vi "Setting Zero Point.vi"(6 "Gas Tank":u8, 7 "Count":u8, 9 "output cluster 3":T2 {"Current Settings"."Pump" items=["Pump 0", "Pump 1", "Pump 2", "Pump 3", "Pump 4", "Pump 5"]; "Current Settings"."Chart X axis Timescale" min=20 max=180 step=1; "Current Settings"."RunTime Mode Settings"."Exp. Gas Tank" items=["0.07", "0.031", "0.877", "1.863", "3.881", "5.790", "7.688", "6.000"]; "Current Settings"."RunTime Mode Settings"."Insp. Gas Tank" items=["0.07", "0.031", "0.877", "1.863", "3.881", "5.790", "7.688", "6.000"]; "Current Settings"."RunTime Mode Settings"."I:E Ratio" max=30 scale=0.0..7.0; "Current Settings"."RunTime Mode Settings"."Resp Rate Brpm" min=0 max=30 format="%.2f"; "Current Settings"."TE#2 Configuration"."Serial Port"."XOFF Char" format="%.0x"; "Current Settings"."TE#2 Configuration"."Serial Port"."XON Char" format="%.0x"; "Current Settings"."TE#2 Configuration"."Serial Port"."flow control" items=["None"=0, "XON/XOFF"=1, "RTS/CTS"=2, "DTR/DSR"=4]; "Current Settings"."TE#2 Configuration"."Serial Port"."stop bits" items=["1.0"=10, "1.5"=15, "2.0"=20]; "Current Settings"."TE#2 Configuration"."Serial Port"."data bits" min=5 max=8 step=1; "Current Settings"."TE#2 Configuration"."Serial Port"."baud rate" items=["75"=75, "110"=110, "134"=134, "150"=150, "300"=300, "600"=600, "1200"=1200, "1800"=1800, "2400"=2400, "4800"=4800, "7200"=7200, "9600"=9600, "14400"=14400, "19200"=19200, "28800"=28800, "38400"=38400, "56000"=56000, "57600"=57600, "115200"=115200, "128000"=128000, "230400"=230400]; "Current Settings"."TE#2 Configuration"."Serial Port"."termination char" format="%.0x"; "Current Settings"."TE#1 Configuration"."Serial Port"."XOFF Char" format="%.0x"; "Current Settings"."TE#1 Configuration"."Serial Port"."XON Char" format="%.0x"; "Current Settings"."TE#1 Configuration"."Serial Port"."flow control" items=["None"=0, "XON/XOFF"=1, "RTS/CTS"=2, "DTR/DSR"=4]; "Current Settings"."TE#1 Configuration"."Serial Port"."stop bits" items=["1.0"=10, "1.5"=15, "2.0"=20]; "Current Settings"."TE#1 Configuration"."Serial Port"."data bits" min=5 max=8 step=1; "Current Settings"."TE#1 Configuration"."Serial Port"."baud rate" items=["75"=75, "110"=110, "134"=134, "150"=150, "300"=300, "600"=600, "1200"=1200, "1800"=1800, "2400"=2400, "4800"=4800, "7200"=7200, "9600"=9600, "14400"=14400, "19200"=19200, "28800"=28800, "38400"=38400, "56000"=56000, "57600"=57600, "115200"=115200, "128000"=128000, "230400"=230400]; "Current Settings"."TE#1 Configuration"."Serial Port"."termination char" format="%.0x"; "Current Settings"."Capnometer Configuration"."Device" items=["None", "TidalWave", "LoFlow / Canary", "Capnogard"]; "Current Settings"."Capnometer Configuration"."Serial Port"."XOFF Char" format="%.0x"; "Current Settings"."Capnometer Configuration"."Serial Port"."XON Char" format="%.0x"; "Current Settings"."Capnometer Configuration"."Serial Port"."flow control" items=["None"=0, "XON/XOFF"=1, "RTS/CTS"=2, "DTR/DSR"=4]; "Current Settings"."Capnometer Configuration"."Serial Port"."stop bits" items=["1.0"=10, "1.5"=15, "2.0"=20]; "Current Settings"."Capnometer Configuration"."Serial Port"."data bits" min=5 max=8 step=1; "Current Settings"."Capnometer Configuration"."Serial Port"."baud rate" items=["75"=75, "110"=110, "134"=134, "150"=150, "300"=300, "600"=600, "1200"=1200, "1800"=1800, "2400"=2400, "4800"=4800, "7200"=7200, "9600"=9600, "14400"=14400, "19200"=19200, "28800"=28800, "38400"=38400, "56000"=56000, "57600"=57600, "115200"=115200, "128000"=128000, "230400"=230400]; "Current Settings"."Capnometer Configuration"."Serial Port"."termination char" format="%.0x"; "Current Settings"."DAQx Settings"."Analog Output Settings (Volts)" format="%#.3g"; "Current Settings"."DAQx Settings"."Duty Cycle" min=10.0 max=90.0 format="%.1g"; "Current Settings"."DAQx Settings"."Frequency" min=20.0 max=200.0; "Current Settings"."DataLogging Settings"."Data File Duration (Minutes)" min=2 max=200 format="%#.2g"; "Current Settings"."Calibration Settings"."Tolerance #2" min=2 max=4096; "Current Settings"."Calibration Settings"."Cal. Average" min=2 max=4096; "Current Settings"."Test Settings"."Test Sensor ID" items=["(select)", "RB", "YC", "", "Other"]}, 10 "CalStatus":T1(ring), 11 "output cluster":T10) -> (2 "NewCalStatus":T1(ring), 3 "Count out":u8)   [LabVIEW 2016]
uses:
  Controls/Cal Refs.ctl
  Controls/DAQ Needed.ctl
  Controls/Processed Variables.ctl
  Controls/AirPump Controls.ctl
  Controls/IE Ratio knob.ctl
  Controls/UI Settings.ctl
  Controls/Aux CO2 Control.ctl
  Controls/Serial Visa Control.ctl
  Controls/Aux CO2 Selector.ctl
  Controls/Aux TE Control.ctl
  Controls/Queues And Others.ctl
  Miscellaneous/Globals.vi
panel:
  # "Note: Setting Brpm to zero will\ndisable Insp / Exp digital output."
  # "mmHg"
  # "pts"
  # "tolerance"
  # "AN5 (Temp 1)"
  # "AN6 (Temp 2)"
  # "AN7 (Temp 3)"
  # "AN8 (T FET)"
  # "AN0 (T POT)"
  # "Tref (Set Pt))"
  # "(Spare)"
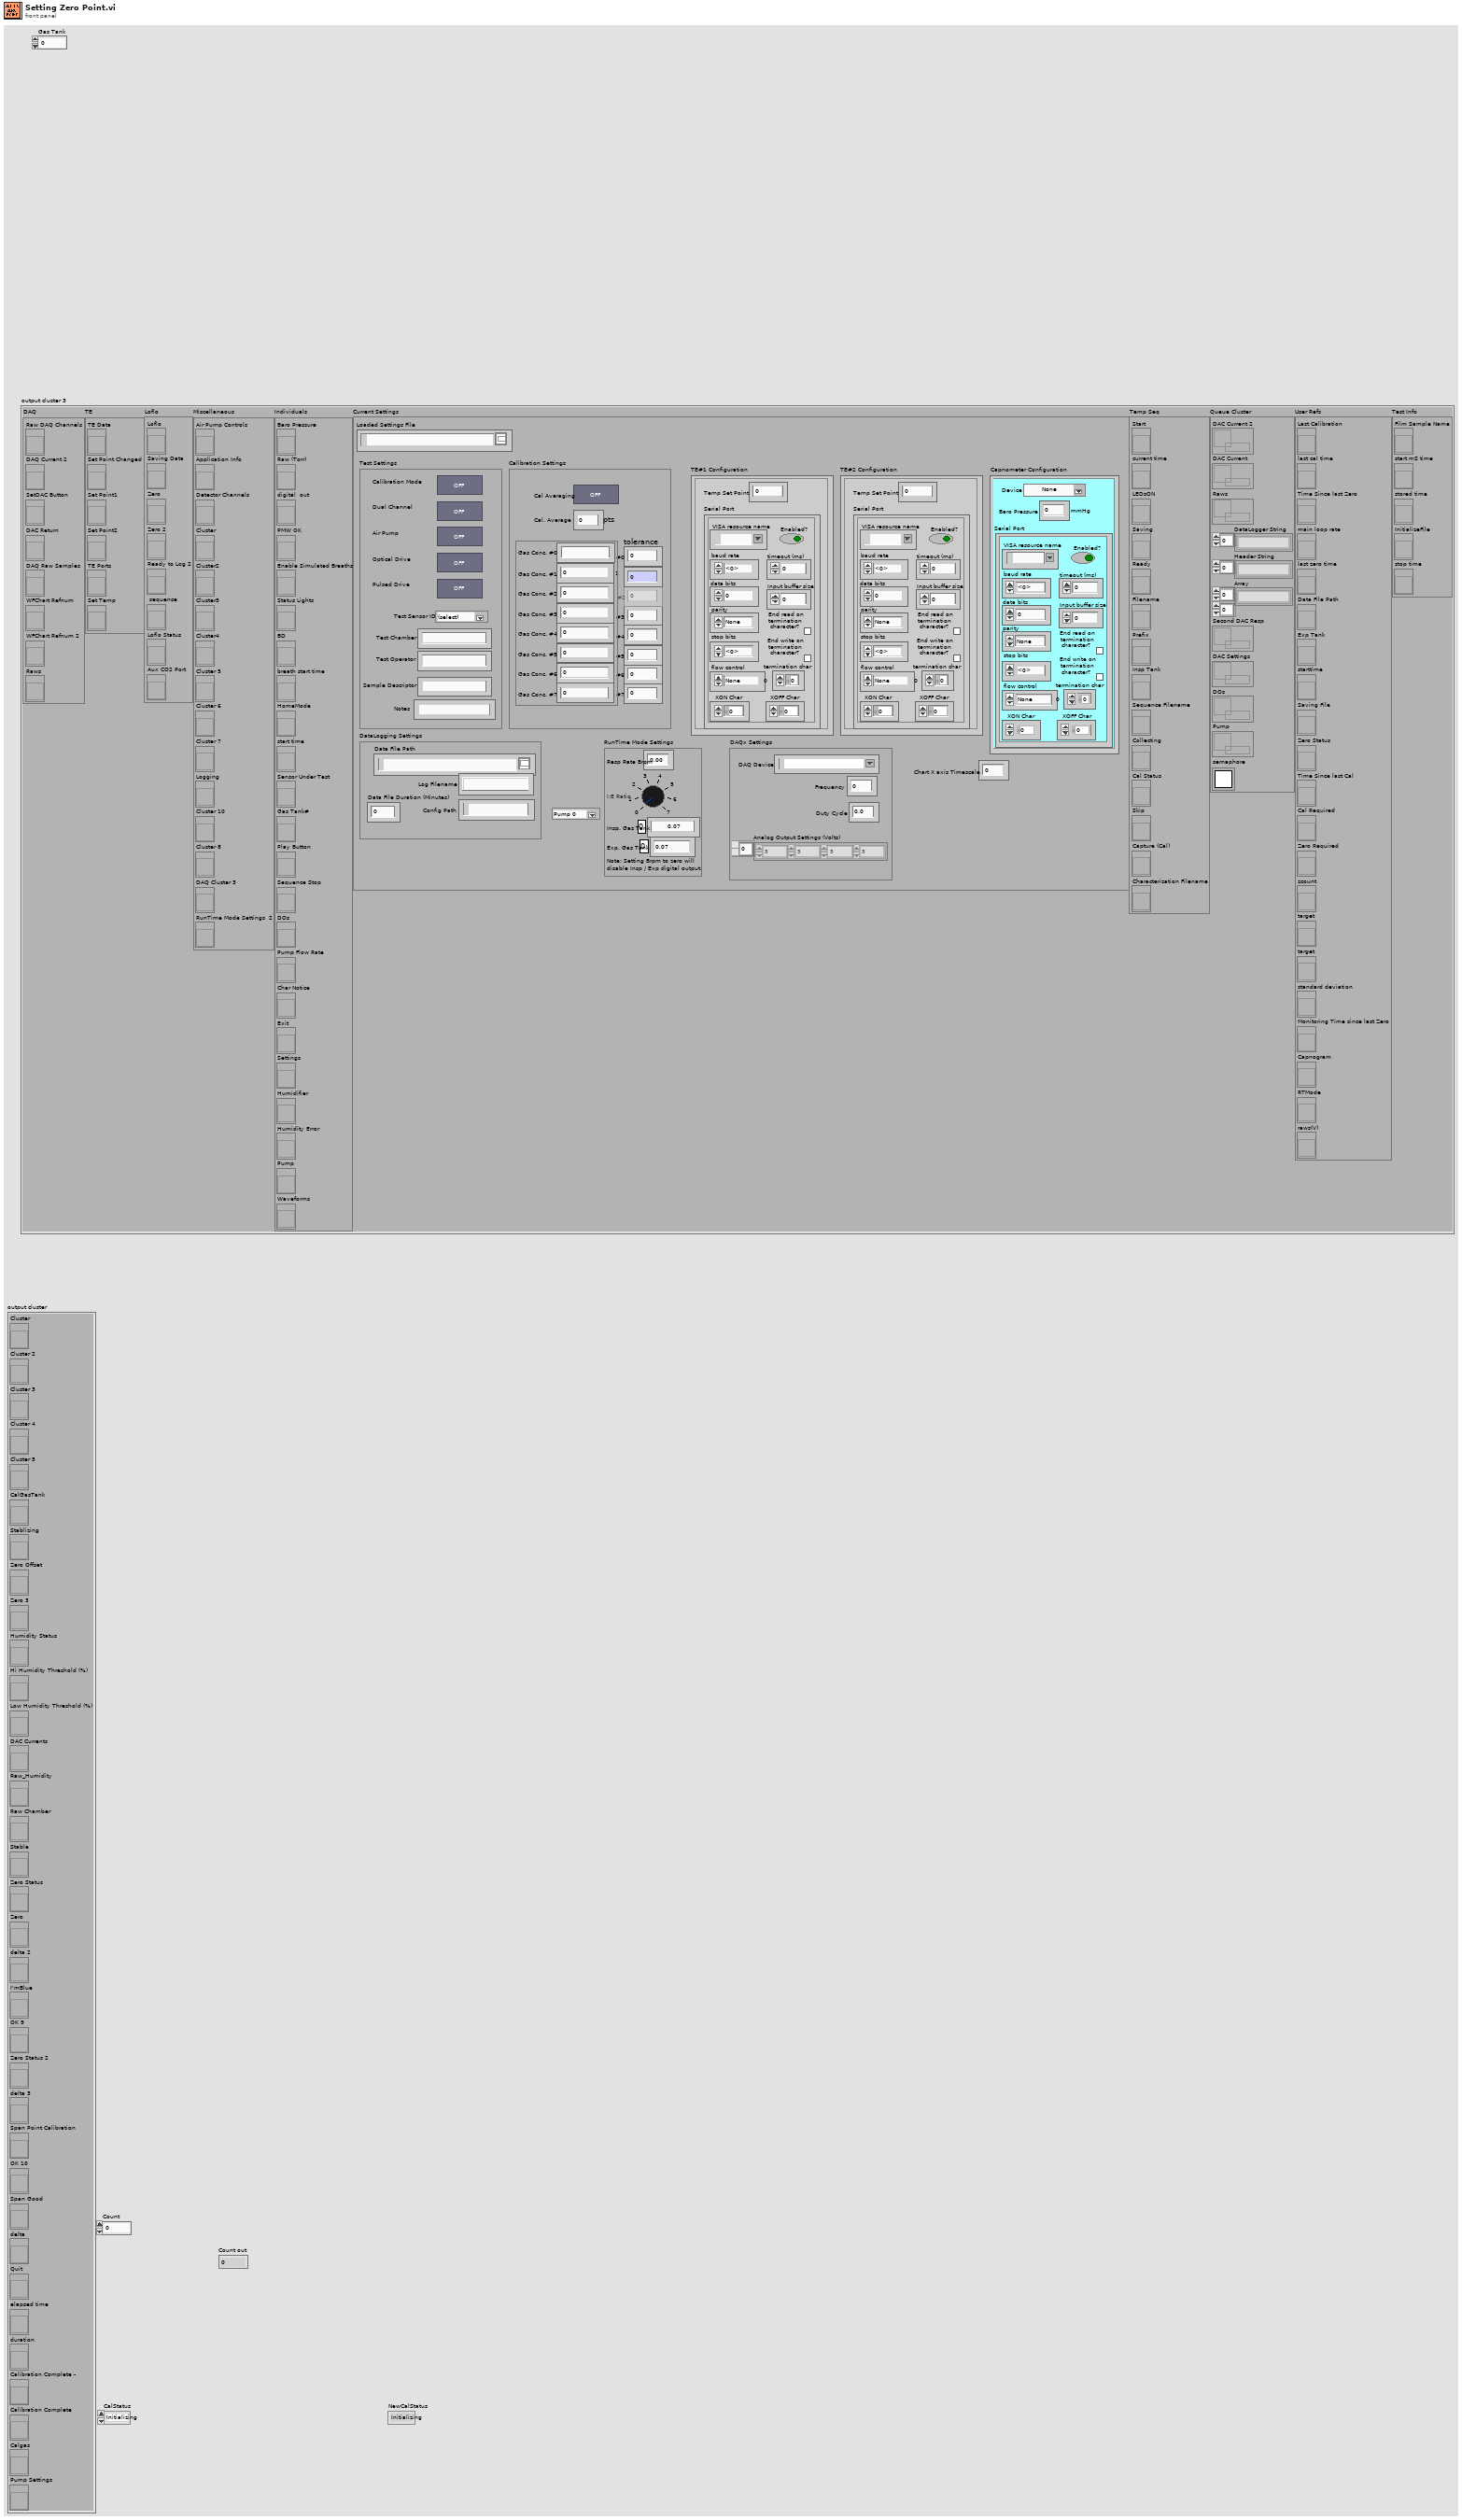
[diagram p1: front panel]
types:
  T1 = enum32{"Initializing", "Enter CO2 Value", "Enter Calibration Code", "Reading Calibration Data", "Stablizing", "Calculating Target Voltages", "Setting Zero Point", "Setting High Point", "Setting Span Point", "Calculating Gain & Offset", "Storing Calibration Coefficients", "Calibration Complete"}
  T2 = typedef "DAQ Needed.ctl" = cluster{"DAQ":cluster{"Raw DAQ Channels":refnum<vi>, "DAQ Current 2":refnum<vi>, "SetDAC Button":refnum<vi>, "DAC Return":refnum<vi>, "DAQ Raw Samples":refnum<vi>, "WFChart Refnum":refnum<vi>, "WFChart Refnum 2":refnum<vi>, "Raws":refnum<vi>}, "TE":cluster{"TE Data":refnum<vi>, "Set Point Changed":refnum<vi>, "Set Point1":refnum<vi>, "Set Point2":refnum<vi>, "TE Ports":refnum<vi>, "Set Temp":refnum<vi>}, "Loflo":cluster{"Loflo":refnum<vi>, "Saving Data":refnum<vi>, "Zero":refnum<vi>, "Zero 2":refnum<vi>, "Ready to Log 2":refnum<vi>, " sequence":refnum<vi>, "Loflo Status ":refnum<vi>, "Aux CO2 Port":refnum<vi>}, "Miscellaneous":cluster{"Air Pump Controls":refnum<vi>, "Application Info":refnum<vi>, "Detector Channels ":refnum<vi>, "Cluster":refnum<vi>, "Cluster2":refnum<vi>, "Cluster3":refnum<vi>, "Cluster4":refnum<vi>, "Cluster 5":refnum<vi>, "Cluster 6":refnum<vi>, "Cluster 7":refnum<vi>, "Logging":refnum<vi>, "Cluster 10":refnum<vi>, "Cluster 8":refnum<vi>, "DAQ Cluster 3":refnum<vi>, "RunTime Mode Settings  2":refnum<vi>}, "Individuals":cluster{"Baro Pressure":refnum<vi>, "Raw (Torr)":refnum<vi>, "digital  out":refnum<vi>, "PMW OK":refnum<vi>, "Enable Simulated Breaths":refnum<vi>, "Status Lights":refnum<vi>, "BD":refnum<vi>, "breath start time":refnum<vi>, "HomeMode":refnum<vi>, "start time":refnum<vi>, "Sensor Under Test":refnum<vi>, "Gas Tank#":refnum<vi>, "Play Button":refnum<vi>, "Sequence Stop":refnum<vi>, "DOs":refnum<vi>, "Pump Flow Rate":refnum<vi>, "Char Notice":refnum<vi>, "Exit":refnum<vi>, "Settings":refnum<vi>, "Humidifier":refnum<vi>, "Humidity Error":refnum<vi>, "Pump":refnum<vi>, "Waveforms":refnum<vi>}, "Current Settings":T3, "Temp Seq":cluster{"Start":refnum<vi>, "current time":refnum<vi>, "LEDsON":refnum<vi>, "Saving":refnum<vi>, "Ready":refnum<vi>, "Filename":refnum<vi>, "Prefix":refnum<vi>, "Insp Tank":refnum<vi>, "Sequence Filename":refnum<vi>, "Collecting":refnum<vi>, "Cal Status":refnum<vi>, "Skip":refnum<vi>, "Capture (Cal)":refnum<vi>, "Characterization Filename":refnum<vi>}, "Queue Cluster":T8, "User Refs":cluster{"Last Calibration":refnum<vi>, "last cal time":refnum<vi>, "Time Since last Zero":refnum<vi>, "main loop rate":refnum<vi>, "last zero time":refnum<vi>, "Data File Path":refnum<vi>, "Exp Tank":refnum<vi>, "starttime":refnum<vi>, "Saving File":refnum<vi>, "Zero Status":refnum<vi>, "Time Since last Cal":refnum<vi>, "Cal Required":refnum<vi>, "Zero Required":refnum<vi>, "zcount":refnum<vi>, "target":refnum<vi>, "target":refnum<vi>, "standard deviation":refnum<vi>, "Monitoring Time since last Zero":refnum<vi>, "Capnogram":refnum<vi>, "RTMode":refnum<vi>, "raws(V)":refnum<vi>}, "Test Info":cluster{"Film Sample Name":refnum<vi>, "start mS time":refnum<vi>, "stored time":refnum<vi>, "InitializeFile":refnum<vi>, "stop time":refnum<vi>}}
  T3 = typedef "UI Settings.ctl" = cluster{"Loaded Settings File":path, "Test Settings":cluster{"Dual Channel":bool, "Air Pump":bool, "Optical Drive":bool, "Pulsed Drive":bool, "Calibration Mode":bool, "Test Sensor ID":u16, "Test Chamber":string, "Test Operator":string, "Sample Descriptor":string, "Notes":string}, "Calibration Settings":cluster{"Cal. Average":u16, "Cal Averaging":bool, "Tolerance #0":sgl, "Tolerance #7":sgl, "Tolerance #6":sgl, "Tolerance #5":sgl, "Tolerance #4":sgl, "Tolerance #3":sgl, "Tolerance #2":sgl, "Tolerance #1":sgl, "Gas Tank Settings":cluster{"Gas Conc. #0":string, "Gas Conc. #1":sgl, "Gas Conc. #2":sgl, "Gas Conc. #3":sgl, "Gas Conc. #4":sgl, "Gas Conc. #5":sgl, "Gas Conc. #6":sgl, "Gas Conc. #7":sgl}}, "DataLogging Settings":cluster{"Data File Path":path, "Data File Duration (Minutes)":sgl, "Log Filename":string, "Config Path":path}, "DAQx Settings":cluster{"DAQ Device":tag, "Frequency":dbl, "Duty Cycle":dbl, "Analog Output Settings (Volts)":sgl[]}, "Capnometer Configuration":T4, "TE#1 Configuration":T7, "TE#2 Configuration":T7, "RunTime Mode Settings ":cluster{"Resp Rate Brpm ":sgl, "I:E Ratio":u8, "Insp. Gas Tank":u16, "Exp. Gas Tank":u16}, "Chart X axis Timescale":u16, "Pump":u16}
  T4 = typedef "Aux CO2 Control.ctl" = cluster{"Serial Port":T5, "Baro Pressure":u32, "Device":T6}
  T5 = typedef "Serial Visa Control.ctl" = cluster{"termination char":u8, "End read on termination character?":bool, "Enabled?":bool, "VISA resource name":refnum<visa-resource-name>, "baud rate":u32, "data bits":u16, "parity":enum16{"None", "Odd", "Even", "Mark", "Space"}, "stop bits":u16, "flow control":u16, "timeout (ms)":u32, "Input buffer size":u32, "End write on termination character?":bool, "XON Char":u8, "XOFF Char":u8}
  T6 = typedef "Aux CO2 Selector.ctl" = u16
  T7 = typedef "Aux TE Control.ctl" = cluster{"Temp Set Point":sgl, "Serial Port":T5}
  T8 = typedef "Queues And Others.ctl" = cluster{"DAC Current 2":refnum<queue>, "DAC Current":refnum<queue>, "Raws":refnum<queue>, "DataLogger String":string[], "Header String":string[], "Array":string[][], "Second DAC Resp":refnum<queue>, "DAC Settings":refnum<queue>, "DOs":refnum<queue>, "Pump":refnum<queue>, "semaphore":T9}
  T9 = typedef "Semaphore RefNum" = refnum<k1>
  T10 = typedef "Cal Refs.ctl" = cluster{"Cluster":refnum<vi>, "Cluster 2":refnum<vi>, "Cluster 3":refnum<vi>, "Cluster 4":refnum<vi>, "Cluster 5":refnum<vi>, "CalGasTank":refnum<vi>, "Stablizing":refnum<vi>, "Zero Offset":refnum<vi>, "Zero 3":refnum<vi>, "Humidity Status":refnum<vi>, "Hi Humidity Threshold (%)":refnum<vi>, "Low Humidity Threshold (%)":refnum<vi>, "DAC Currents":refnum<vi>, "Raw_Humidity":refnum<vi>, "Raw Chamber":refnum<vi>, "Stable":refnum<vi>, "Zero Status":refnum<vi>, "Zero":refnum<vi>, "delta 2":refnum<vi>, "I'mBlue":refnum<vi>, "OK 9":refnum<vi>, "Zero Status 2":refnum<vi>, "delta 3":refnum<vi>, "Span Point Calibration":refnum<vi>, "OK 10":refnum<vi>, "Span Good":refnum<vi>, "delta":refnum<vi>, "Quit":refnum<vi>, "elapsed time":refnum<vi>, "duration":refnum<vi>, "Calibration Complete -":refnum<vi>, "Calibration Complete":refnum<vi>, "Calgas":refnum<vi>, "Pump Settings":refnum<vi>}
  T11 = cluster{"Tcal_Chamber":dbl, "Tcal_PCB":dbl, "Tcal_Film":dbl, "Tcal_Humidity":dbl, "Tcal_Det":dbl[], "Cal Gas":dbl, "Reference":dbl}
  T12 = enum16{"Setting Zero at 5 mA", "Setting Zero at 15 mA", "Calculating slopes"}
  T13 = cluster{"CHANNEL 2":string[], "BlueLED":bool[], "V_RA(5mA)":dbl[], "V_RA(15mA)":dbl[], "mI":dbl[], "DAC scale":dbl[]}
  T14 = cluster{"CalFile Selected":path, "TYPE":string, "DATE":string, "C0FC2V":dbl[], "C6FC2V":dbl[], "V_0d(target)":dbl[], "V_6d(target)":dbl[], "V_span(target)":dbl[], "CHANNEL":string[], "Status":bool[], "BlueLED 2":bool[], "C2V":u8[], "A":dbl[], "B":dbl[], "C":dbl[], "D":dbl[], "V2C":u8[], "A'":dbl[], "B'":dbl[], "C'":dbl[], "D'":dbl[]}
  T15 = typedef "Calibration Coefficients.ctl" = cluster{"CalFile Used":path, "TYPE":string, "DATE":string, "Humidity":sgl, "Chamber Temp":dbl, "CO2_calgas":dbl, "V_(RA,5mA)":dbl, "V_(RA,15mA)":dbl, "mI":dbl, "V_0d_ImA (actual)":dbl, "V_6d_ImA (actual)":dbl, "I_span":dbl, "DAC":u16, "A":dbl, "B":dbl, "C":dbl, "D":dbl, "V6d":dbl, "A'":dbl, "B'":dbl, "C'":dbl, "D'":dbl, "V0d":dbl, "CalDate":string, "CalTime":string, "duration":dbl, "Detector Channel":string, "a2":dbl, "a3":dbl, "a4":dbl, "a5":dbl, "b2":dbl, "c2":dbl, "b3":dbl, "c3":dbl, "b4":dbl, "c4":dbl, "b5":dbl, "c5":dbl, "a7":dbl, "a8":dbl, "a9":dbl, "a10":dbl, "b7":dbl, "b8":dbl, "b9":dbl, "b10":dbl, "c7":dbl, "c8":dbl, "c9":dbl, "c10":dbl, "cal_offs_adj":dbl, "cal_gain_adj":dbl, "C6d":dbl, "C0d":dbl, "Cal_currernt":dbl, "C2V":u16, "V2C":u16, "Zero Date":string, "Zero Time":string, "Number of Zeroes":u16, "V_(()d, average)":dbl, "V_offs ":dbl, "G_adj":dbl, "Pump Flow Rate":u16, "Zero Required? ":bool, "Calibrate Required?":bool, "cal_utc":dbl, "zero_utc":dbl, "Elapsed Time":dbl, "PCB":string, "m0":dbl, "b0":dbl}
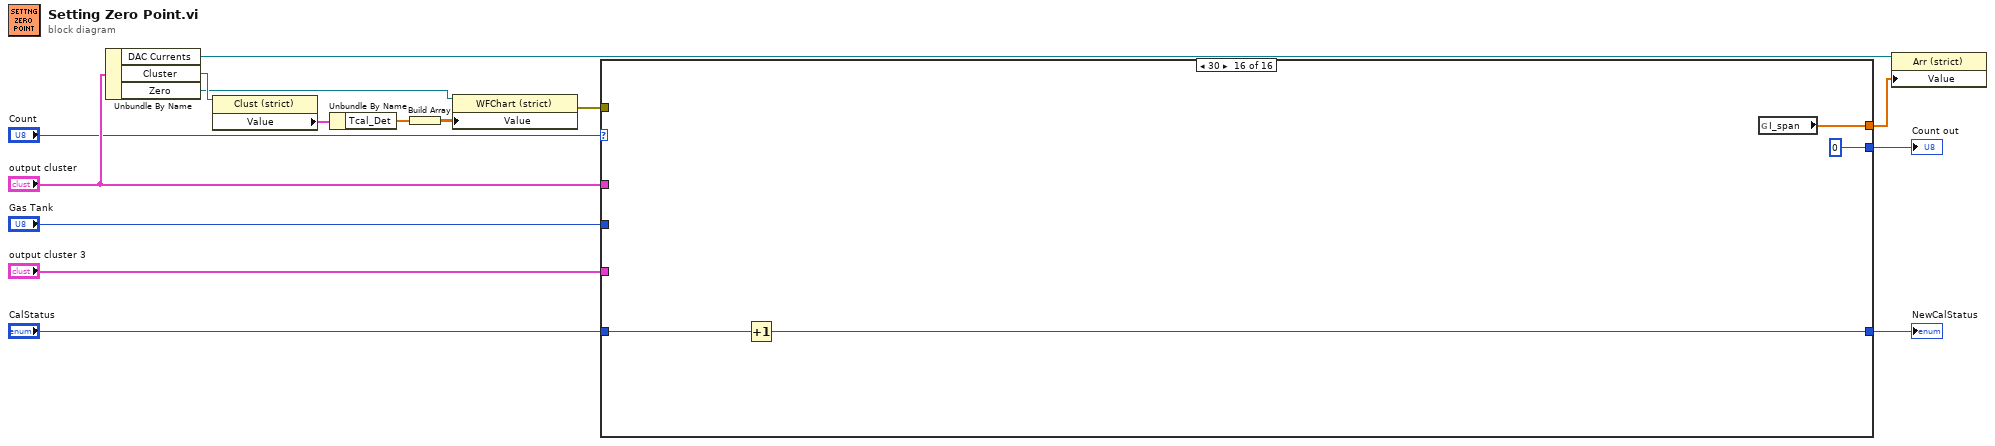
[diagram p0: block diagram]
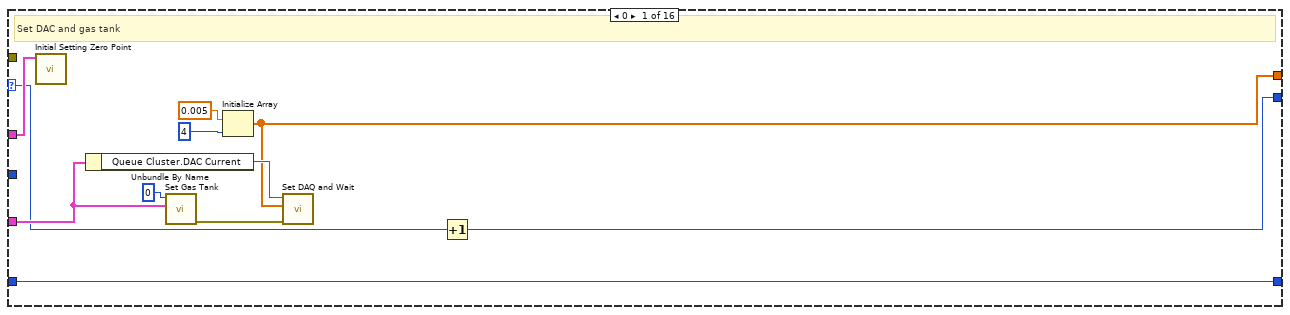
[diagram p2: hidden frame]
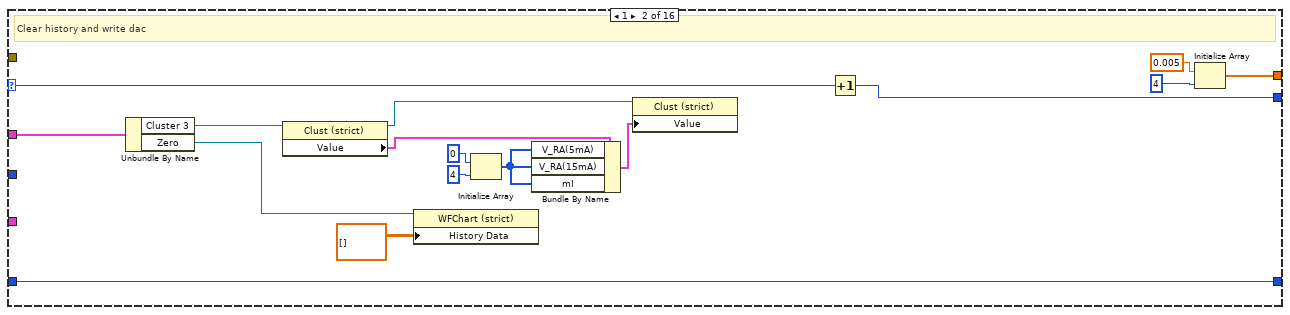
[diagram p3: hidden frame]
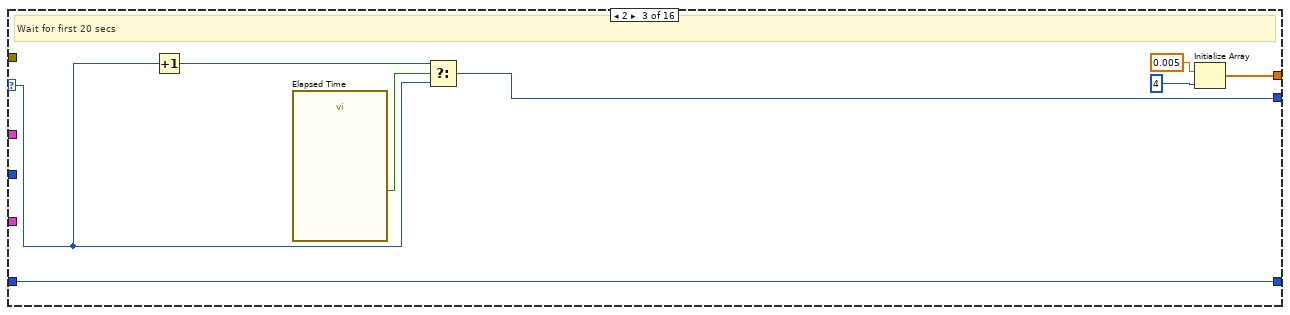
[diagram p4: hidden frame]
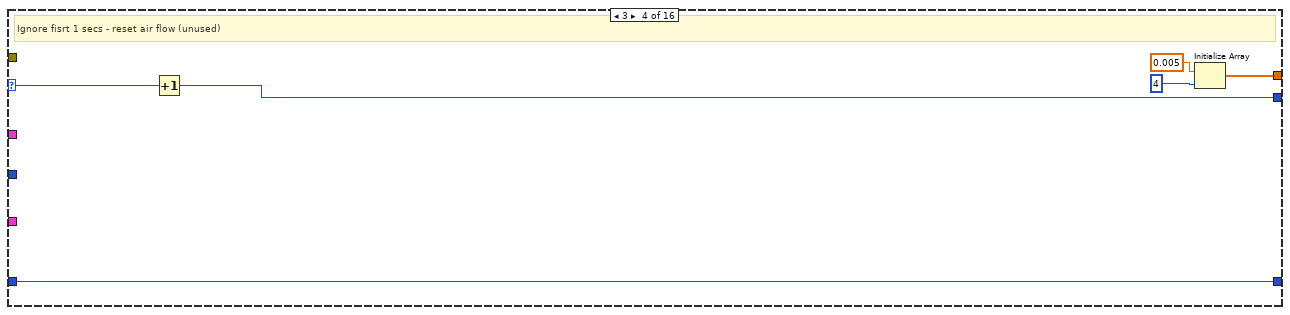
[diagram p5: hidden frame]
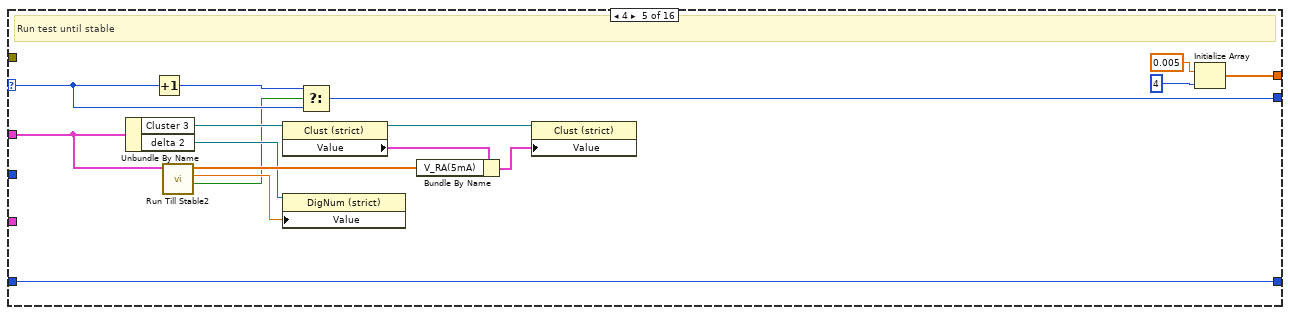
[diagram p6: hidden frame]
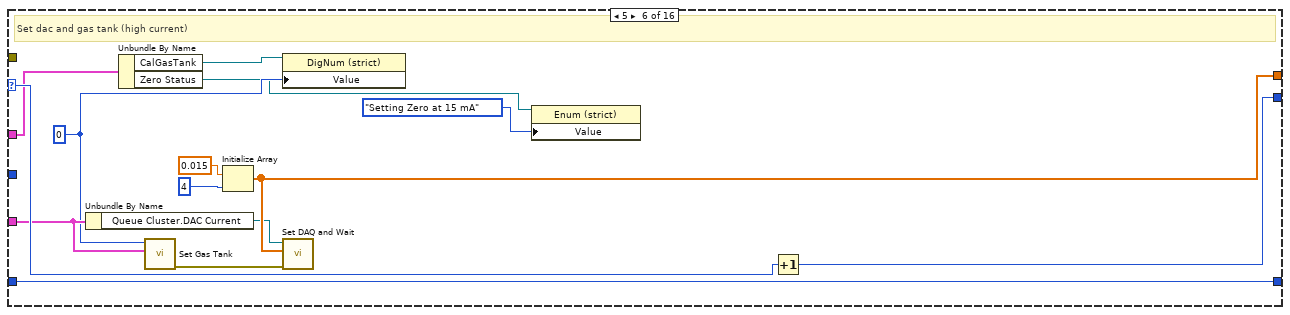
[diagram p7: hidden frame]
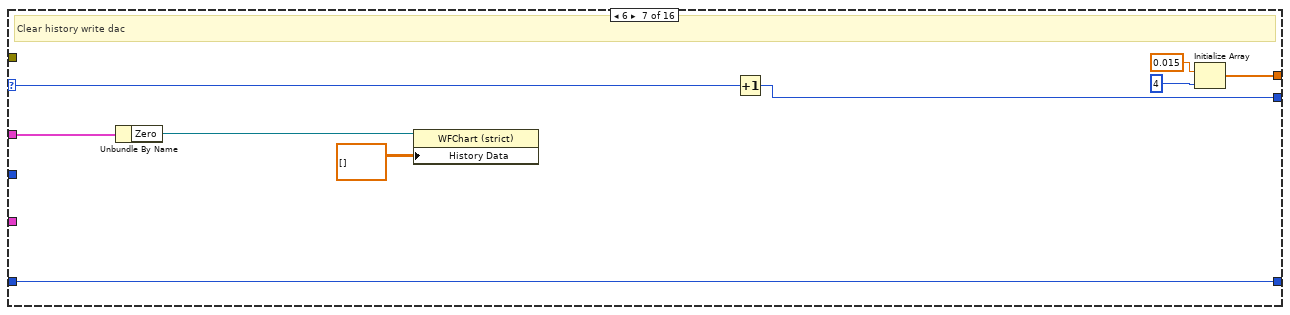
[diagram p8: hidden frame]
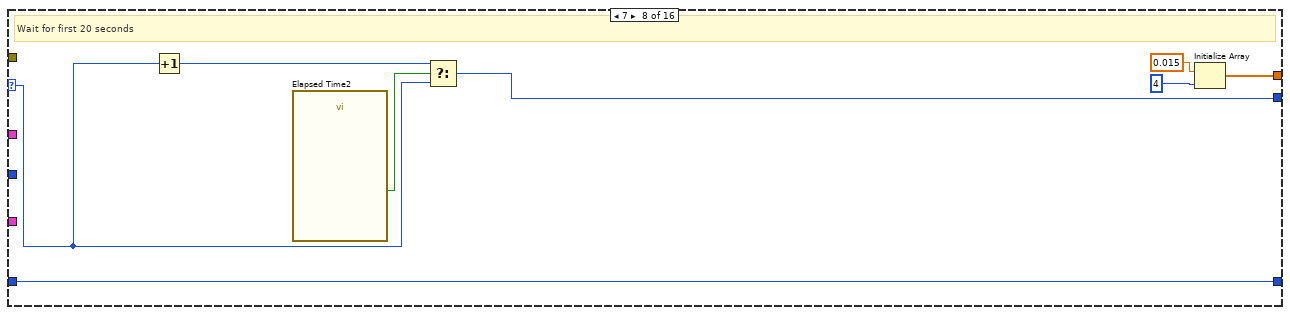
[diagram p9: hidden frame]
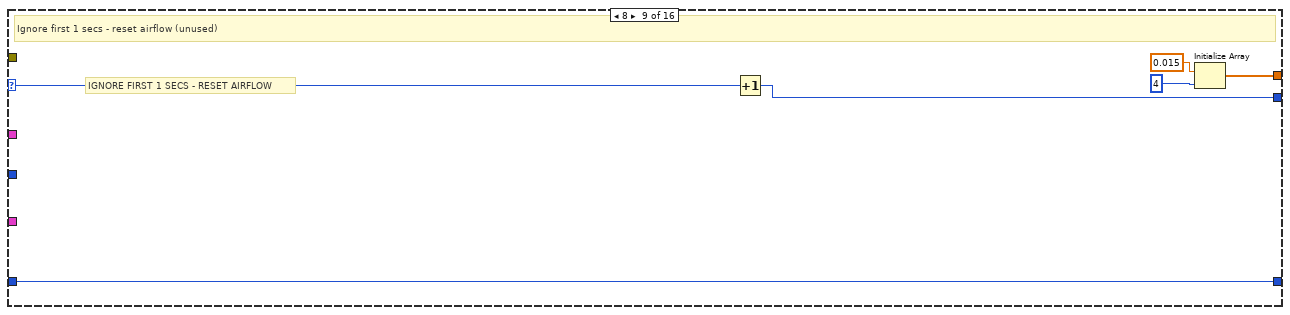
[diagram p10: hidden frame]
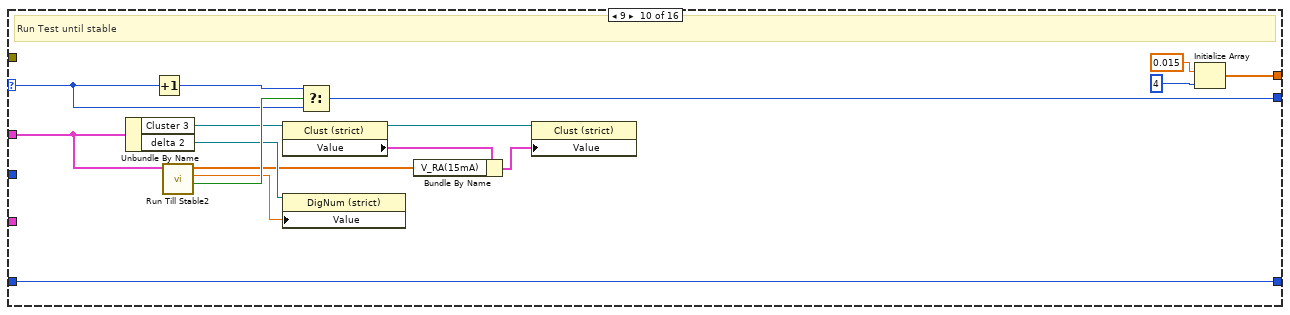
[diagram p11: hidden frame]
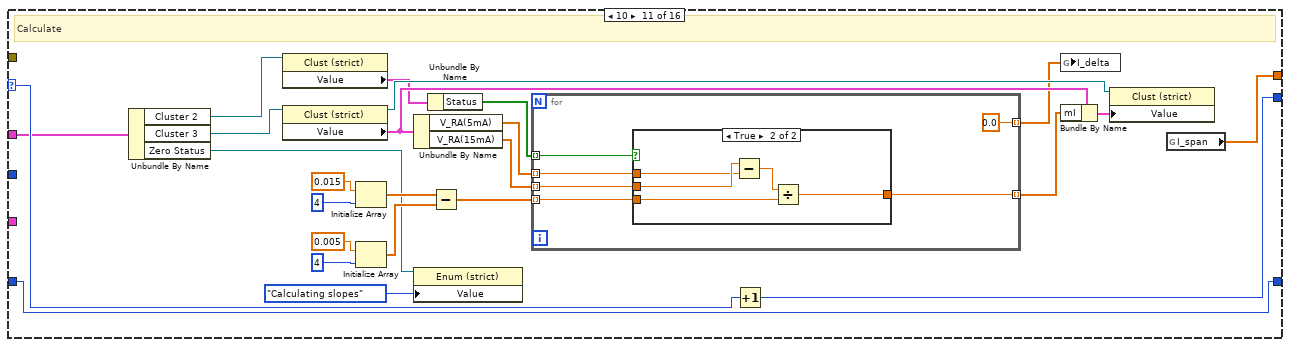
[diagram p12: hidden frame]
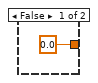
[diagram p13: hidden frame]
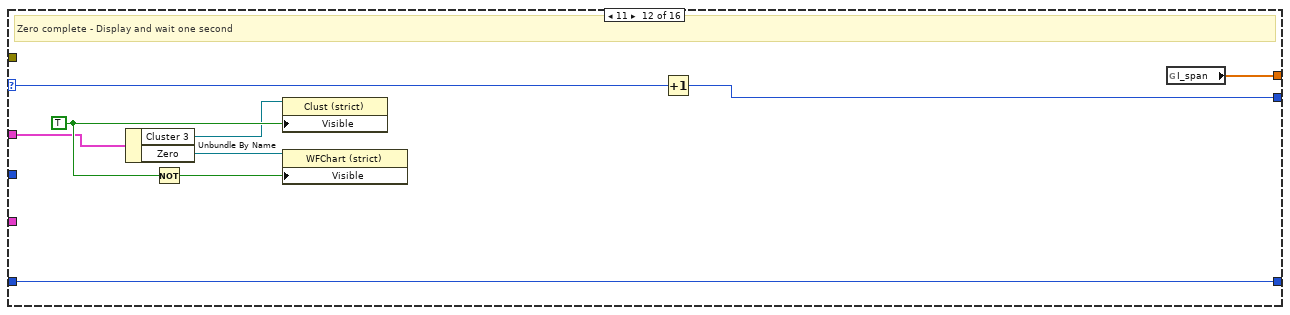
[diagram p14: hidden frame]
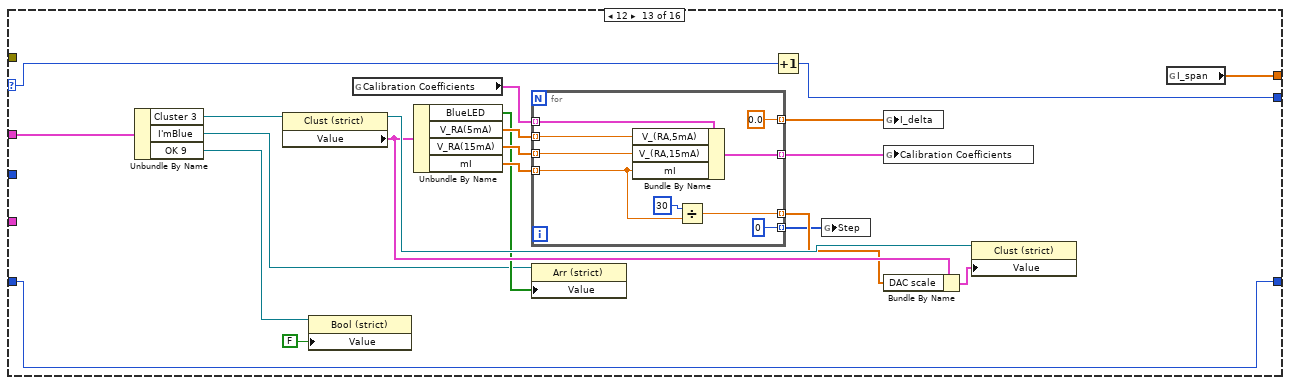
[diagram p15: hidden frame]
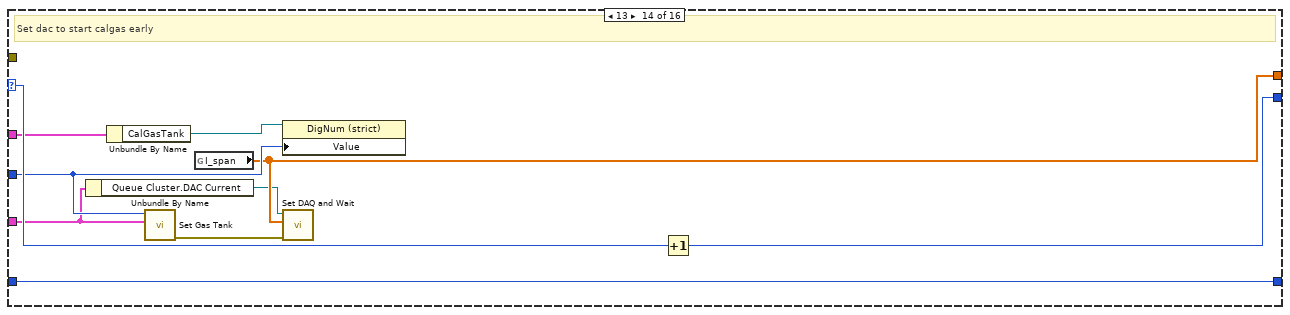
[diagram p16: hidden frame]
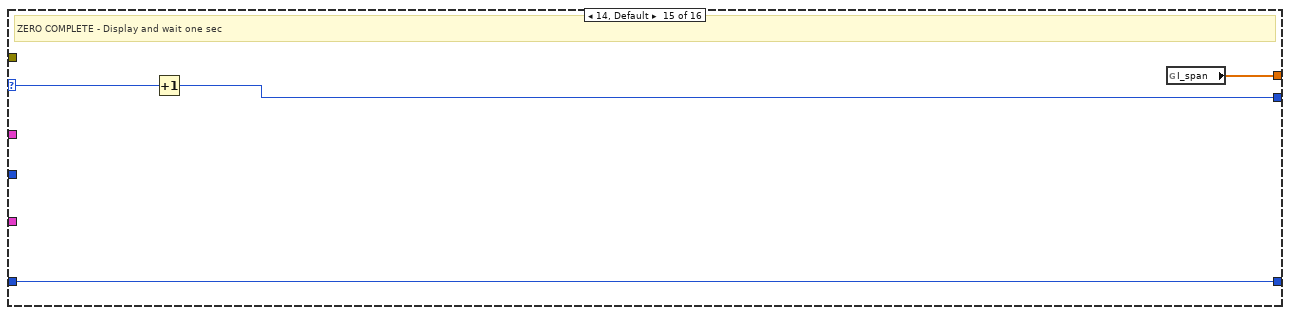
[diagram p17: hidden frame]
diagram:
  n1 = Unbundle By Name("output cluster") -> ("DAC Currents"=w13:refnum<vi>, "Cluster"=w11:refnum<vi>, "Zero"=w8:refnum<vi>)
  n2 = property class="Clust (strict)"(reference=w11) -> ("Value"=w10:T11)  [unwired: 1 in, 2 out]
  n3 = Unbundle By Name(w10) -> ("Tcal_Det"=w9:dbl[])
  n4 = Build Array(w9) -> (w7:dbl[][])
  n5 = property class="WFChart (strict)"(reference=w8, "Value"=w7) -> (error out=w6:errorcluster)  [unwired: 1 in, 1 out]
  n6 = case shown="30" "Count" {
    selector: "Count" -> [w17 w42 w50 w56 w70 w86 w95 w103 w109 w122 w148 w170 w191 w210 w214 _]
    tunnel: [w16 w41 w48 w54 w69 w85 w94 w101 w107 w123 w149 w169 w190 w209 w213 0] -> w2
    tunnel: "CalStatus" -> [w26 w40 w47 w55 w71 w84 w93 w100 w108 w125 w150 w171 w189 w211 w215 w218]
    tunnel: [w26 w40 w47 w55 w71 w84 w93 w100 w108 w125 w150 w171 w189 w211 w215 w217] -> w3
    tunnel: [w21 w28 w44 w51 w66 w75 w89 w97 w104 w118 w134 w166 w177 w205 w212 w216] -> w12
    tunnel: "Gas Tank" -> [_ _ _ _ _ _ _ _ _ _ _ _ _ w208 _ _]
    tunnel: "output cluster 3" -> [w23 _ _ _ _ w79 _ _ _ _ _ _ _ w206 _ _]
    tunnel: "output cluster" -> [w19 w32 _ _ w65 w83 w88 _ _ w117 w140 w165 w181 w203 _ _]
    tunnel: w6 -> [_ _ _ _ _ _ _ _ _ _ _ _ _ _ _ _]
    frame 0 {
      # "Set DAC and gas tank"
      n7 = call "Initial Setting Zero Point.vi"("output cluster"=w19) -> ()  [unwired: 11 in]
      n8 = Unbundle By Name(w23) -> ("Queue Cluster.DAC Current"=w22:refnum<queue>)
      n9 = call "Set Gas Tank.vi"("input cluster"=w23, "Gas Tank"=u8 0 ("CalGasTank")) -> ("error out"=w18:errorcluster)  [unwired: 8 in, 1 out]
      n10 = Initialize Array(0.005, 4 ("index")) -> (w21:dbl[])
      n11 = call "Set DAQ and Wait.vi"("error in (no error)"=w18, "Array"=w21, "Queue in"=w22) -> ()  [unwired: 9 in]
      n12 = Increment(x=w17) -> (x+1=w16:u8)
    }
    frame 1 {
      # "Clear history and write dac"
      n13 = Unbundle By Name(w32) -> ("Cluster 3"=w31:refnum<vi>, "Zero"=w27:refnum<vi>)
      n14 = property class="Clust (strict)"(reference=w31) -> (reference out=w36:refnum<vi>, "Value"=w35:T13)  [unwired: 1 in, 1 out]
      n15 = property on="Property Node" class="WFChart (strict)"(reference=w27, "History Data"=dbl[][] []) -> ()  [unwired: 1 in, 2 out]
      n16 = Initialize Array(0, 4 ("dimension size")) -> (w33:i32[])
      n17 = Bundle By Name(cluster=w35, "V_RA(5mA)"=w33, "V_RA(15mA)"=w33, "mI"=w33) -> (w34:T13)
      n18 = property class="Clust (strict)"(reference=w36, "Value"=w34) -> ()  [unwired: 1 in, 2 out]
      n19 = Increment(x=w42) -> (x+1=w41:u8)
      n20 = Initialize Array(0.005, 4 ("index")) -> (w28:dbl[])
    }
    frame 2 {
      # "Wait for first 20 secs"
      n21 = Increment(x=w50) -> (x+1=w49:u8)
      n22 = call "Elapsed Time"() -> ("Time has Elapsed"=w43:bool)  [unwired: 12 in, 7 out]
      n23 = Select(t=w49, s=w43, f=w50) -> (s? t:f=w48:u8)
      n24 = Initialize Array(0.005, 4 ("index")) -> (w44:dbl[])
    }
    frame 3 {
      # "Ignore fisrt 1 secs - reset air flow (unused)"
      n25 = Increment(x=w56) -> (x+1=w54:u8)
      n26 = Initialize Array(0.005, 4 ("index")) -> (w51:dbl[])
    }
    frame 4 {
      # "Run test until stable"
      n27 = Unbundle By Name(w65) -> ("Cluster 3"=w64:refnum<vi>, "delta 2"=w59:refnum<vi>)
      n28 = Increment(x=w70) -> (x+1=w72:u8)
      n29 = call "Run Till Stable2.vi"("output cluster"=w65) -> ("Boolean"=w57:bool, "Delta"=w58:dbl, "Array"=w63:dbl[])  [unwired: 8 in]
      n30 = property class="Clust (strict)"(reference=w64) -> (reference out=w62:refnum<vi>, "Value"=w61:T13)  [unwired: 1 in, 1 out]
      n31 = property class="DigNum (strict)"(reference=w59, "Value"=w58) -> ()  [unwired: 1 in, 2 out]
      n32 = Select(t=w72, s=w57, f=w70) -> (s? t:f=w69:u8)
      n33 = Bundle By Name(cluster=w61, "V_RA(5mA)"=w63) -> (w60:T13)
      n34 = property class="Clust (strict)"(reference=w62, "Value"=w60) -> ()  [unwired: 1 in, 2 out]
      n35 = Initialize Array(0.005, 4 ("index")) -> (w66:dbl[])
    }
    frame 5 {
      w78 = u8 0 ("CalGasTank")
      # "Set dac and gas tank (high current)"
      n36 = Unbundle By Name(w79) -> ("Queue Cluster.DAC Current"=w74:refnum<queue>)
      n37 = Unbundle By Name(w83) -> ("CalGasTank"=w82:refnum<vi>, "Zero Status"=w73:refnum<vi>)
      n38 = call "Set Gas Tank.vi"("input cluster"=w79, "Gas Tank"=w78) -> ("error out"=w76:errorcluster)  [unwired: 8 in, 1 out]
      n39 = Initialize Array(0.015, 4 ("index")) -> (w75:dbl[])
      n40 = property class="DigNum (strict)"(reference=w82, "Value"=w78) -> ()  [unwired: 1 in, 2 out]
      n41 = call "Set DAQ and Wait.vi"("error in (no error)"=w76, "Array"=w75, "Queue in"=w74) -> ()  [unwired: 9 in]
      n42 = property class="Enum (strict)"(reference=w73, "Value"=T12."Setting Zero at 15 mA" ("Zero Status")) -> ()  [unwired: 1 in, 2 out]
      n43 = Increment(x=w86) -> (x+1=w85:u8)
    }
    frame 6 {
      # "Clear history write dac"
      n44 = Unbundle By Name(w88) -> ("Zero"=w87:refnum<vi>)
      n45 = property on="Property Node" class="WFChart (strict)"(reference=w87, "History Data"=dbl[][] []) -> ()  [unwired: 1 in, 2 out]
      n46 = Increment(x=w95) -> (x+1=w94:u8)
      n47 = Initialize Array(0.015, 4 ("index")) -> (w89:dbl[])
    }
    frame 7 {
      # "Wait for first 20 seconds"
      n48 = Increment(x=w103) -> (x+1=w102:u8)
      n49 = call "Elapsed Time2"() -> ("Time has Elapsed"=w96:bool)  [unwired: 12 in, 7 out]
      n50 = Select(t=w102, s=w96, f=w103) -> (s? t:f=w101:u8)
      n51 = Initialize Array(0.015, 4 ("index")) -> (w97:dbl[])
    }
    frame 8 {
      # "IGNORE FIRST 1 SECS - RESET AIRFLOW"
      # "Ignore first 1 secs - reset airflow (unused)"
      n52 = Increment(x=w109) -> (x+1=w107:u8)
      n53 = Initialize Array(0.015, 4 ("index")) -> (w104:dbl[])
    }
    frame 9 {
      # "Run Test until stable"
      n54 = Unbundle By Name(w117) -> ("Cluster 3"=w116:refnum<vi>, "delta 2"=w112:refnum<vi>)
      n55 = Increment(x=w122) -> (x+1=w121:u8)
      n56 = call "Run Till Stable2.vi"("output cluster"=w117) -> ("Boolean"=w124:bool, "Delta"=w110:dbl, "Array"=w111:dbl[])  [unwired: 8 in]
      n57 = property class="Clust (strict)"(reference=w116) -> (reference out=w113:refnum<vi>, "Value"=w115:T13)  [unwired: 1 in, 1 out]
      n58 = property class="DigNum (strict)"(reference=w112, "Value"=w110) -> ()  [unwired: 1 in, 2 out]
      n59 = Select(t=w121, s=w124, f=w122) -> (s? t:f=w123:u8)
      n60 = Bundle By Name(cluster=w115, "V_RA(15mA)"=w111) -> (w114:T13)
      n61 = property class="Clust (strict)"(reference=w113, "Value"=w114) -> ()  [unwired: 1 in, 2 out]
      n62 = Initialize Array(0.015, 4 ("index")) -> (w118:dbl[])
    }
    frame 10 {
      # "Calculate"
      n63 = Unbundle By Name(w140) -> ("Cluster 2"=w138:refnum<vi>, "Cluster 3"=w139:refnum<vi>, "Zero Status"=w126:refnum<vi>)
      n64 = property class="Clust (strict)"(reference=w138) -> ("Value"=w137:T14)  [unwired: 1 in, 2 out]
      n65 = property class="Clust (strict)"(reference=w139) -> (reference out=w144:refnum<vi>, "Value"=w143:T13)  [unwired: 1 in, 1 out]
      n66 = Initialize Array(0.015, 4 ("index")) -> (w131:dbl[])
      n67 = Initialize Array(0.005, 4 ("index")) -> (w128:dbl[])
      n68 = Unbundle By Name(w143) -> ("V_RA(5mA)"=w146:dbl[], "V_RA(15mA)"=w145:dbl[])
      n69 = property class="Enum (strict)"(reference=w126, "Value"=T12."Calculating slopes" ("Zero Status")) -> ()  [unwired: 1 in, 2 out]
      n70 = Unbundle By Name(w137) -> ("Status"=w136:bool[])
      n71 = Subtract(x=w131, y=w128) -> (x-y=w147:dbl[])
      n72 = for {
        tunnel: w147 -> [w154] mode=indexing
        tunnel: w146 -> [w155] mode=indexing
        tunnel: w145 -> [w156] mode=indexing
        tunnel: [w153] -> w141 mode=indexing
        tunnel: [0.0 ("x*y")] -> w135 mode=indexing
        tunnel: w136 -> [w151] mode=indexing
        n73 = case shown="True" w151 {
          tunnel: w156 -> [_ w162]
          tunnel: w155 -> [_ w161]
          tunnel: w154 -> [_ w159]
          tunnel: [0.0 w158] -> w153
          frame False {
          }
          frame True {
            n74 = Subtract(x=w162, y=w161) -> (x-y=w160:dbl)
            n75 = Divide(x=w160, y=w159) -> (x/y=w158:dbl)
          }
        }
      }
      n76 = Increment(x=w148) -> (x+1=w149:u8)
      n77 = global write "Globals.vi" "I_delta"(w135) -> ()
      n78 = Bundle By Name(cluster=w143, "mI"=w141) -> (w142:T13)
      n79 = property class="Clust (strict)"(reference=w144, "Value"=w142) -> ()  [unwired: 1 in, 2 out]
      n80 = global read "Globals.vi" "I_span"() -> (w134:dbl[])
    }
    frame 11 {
      w167 = TRUE ("Visible")
      # "Zero complete - Display and wait one second"
      n81 = Unbundle By Name(w165) -> ("Cluster 3"=w164:refnum<vi>, "Zero"=w163:refnum<vi>)
      n82 = Not(x=w167) -> (.not. x?=w168:bool)
      n83 = property on="Property Node" class="Clust (strict)"(reference=w164, "Visible"=w167) -> ()  [unwired: 1 in, 2 out]
      n84 = property on="Property Node" class="WFChart (strict)"(reference=w163, "Visible"=w168) -> ()  [unwired: 1 in, 2 out]
      n85 = Increment(x=w170) -> (x+1=w169:u8)
      n86 = global read "Globals.vi" "I_span"() -> (w166:dbl[])
    }
    frame 12 {
      n87 = Unbundle By Name(w181) -> ("Cluster 3"=w180:refnum<vi>, "I'mBlue"=w175:refnum<vi>, "OK 9"=w174:refnum<vi>)
      n88 = property class="Clust (strict)"(reference=w180) -> (reference out=w185:refnum<vi>, "Value"=w184:T13)  [unwired: 1 in, 1 out]
      n89 = property class="Bool (strict)"(reference=w174, "Value"=FALSE) -> ()  [unwired: 1 in, 2 out]
      n90 = global read "Globals.vi" "Calibration Coefficients"() -> (w173:T15[])
      n91 = Unbundle By Name(w184) -> ("BlueLED"=w176:bool[], "V_RA(5mA)"=w188:dbl[], "V_RA(15mA)"=w187:dbl[], "mI"=w186:dbl[])
      n92 = for {
        tunnel: w186 -> [w194] mode=indexing
        tunnel: w173 -> [w201] mode=indexing
        tunnel: [w200] -> w172 mode=indexing
        tunnel: w188 -> [w199] mode=indexing
        tunnel: w187 -> [w198] mode=indexing
        tunnel: [0.0] -> w179 mode=indexing
        tunnel: [i8 0 ("Step")] -> w178 mode=indexing
        tunnel: [w193] -> w183 mode=indexing
        n93 = Bundle By Name(cluster=w201, "V_(RA,5mA)"=w199, "V_(RA,15mA)"=w198, "mI"=w194) -> (w200:T15)
        n94 = Divide(x=30, y=w194) -> (x/y=w193:dbl)
      }
      n95 = property class="Arr (strict)"(reference=w175, "Value"=w176) -> ()  [unwired: 1 in, 2 out]
      n96 = Increment(x=w191) -> (x+1=w190:u8)
      n97 = global write "Globals.vi" "Step"(w178) -> ()
      n98 = global write "Globals.vi" "I_delta"(w179) -> ()
      n99 = global write "Globals.vi" "Calibration Coefficients"(w172) -> ()
      n100 = Bundle By Name(cluster=w184, "DAC scale"=w183) -> (w182:T13)
      n101 = property class="Clust (strict)"(reference=w185, "Value"=w182) -> ()  [unwired: 1 in, 2 out]
      n102 = global read "Globals.vi" "I_span"() -> (w177:dbl[])
    }
    frame 13 {
      # "Set dac to start calgas early"
      n103 = Unbundle By Name(w206) -> ("Queue Cluster.DAC Current"=w204:refnum<queue>)
      n104 = Unbundle By Name(w203) -> ("CalGasTank"=w207:refnum<vi>)
      n105 = call "Set Gas Tank.vi"("input cluster"=w206, "Gas Tank"=w208) -> ("error out"=w202:errorcluster)  [unwired: 8 in, 1 out]
      n106 = global read "Globals.vi" "I_span"() -> (w205:dbl[])
      n107 = property class="DigNum (strict)"(reference=w207, "Value"=w208) -> ()  [unwired: 1 in, 2 out]
      n108 = call "Set DAQ and Wait.vi"("error in (no error)"=w202, "Array"=w205, "Queue in"=w204) -> ()  [unwired: 9 in]
      n109 = Increment(x=w210) -> (x+1=w209:u8)
    }
    frame 14, Default {
      # "ZERO COMPLETE - Display and wait one sec"
      n110 = Increment(x=w214) -> (x+1=w213:u8)
      n111 = global read "Globals.vi" "I_span"() -> (w212:dbl[])
    }
    frame 30 {
      n112 = Increment(x=w218) -> (x+1=w217:T1)
      n113 = global read "Globals.vi" "I_span"() -> (w216:dbl[])
    }
  }
  "NewCalStatus" <- w3
  "Count out" <- w2
  n114 = property class="Arr (strict)"(reference=w13, "Value"=w12) -> ()  [unwired: 1 in, 2 out]
